vi "Angle.vi"() -> ()   [LabVIEW 2013]
uses:
  Robot Global Data.vi
panel:
  out "Angle":dbl
  in  "Samples Per Second":dbl=1000.0
  in  "Average Bits":u8=3 max=15
  out "Voltage Display":cluster{"Value":dbl, "Voltage":dbl}(graph)
  out "Average Voltage":dbl
  out "Voltage":dbl
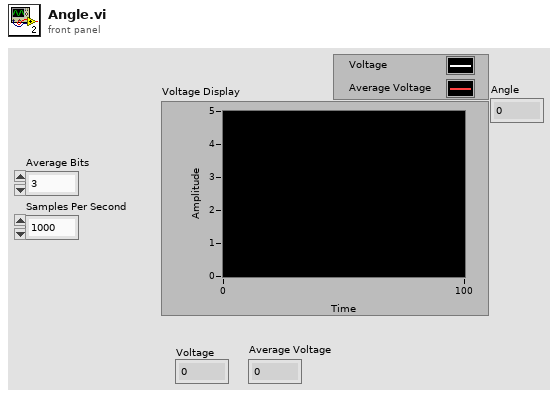
[diagram p1: front panel]
types:
  T1 = typedef "WPI_AnalogChannelDevRef.ctl" = cluster{"DevStatus":errorcluster, "Analog Module":T2, "Analog Channel":T3}
  T2 = typedef "FPGA_TypedefAnalogModule.ctl" = enum16{"Analog Module 1", "Analog Module 2"}
  T3 = typedef "FPGA_AIChannel.ctl" = enum8{"AI 1", "AI 2", "AI 3", "AI 4", "AI 5", "AI 6", "AI 7", "AI 8", "Invalid"}
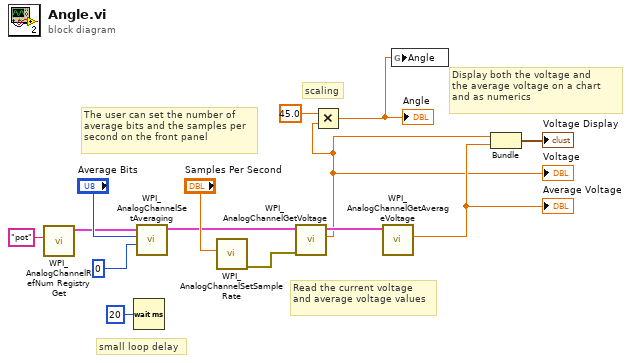
[diagram p0: block diagram]
diagram:
  # "scaling"
  # "small loop delay"
  # "Read the current voltage\nand average voltage values"
  # "Display both the voltage and\nthe average voltage on a chart\nand as numerics"
  # "The user can set the number of \naverage bits and the samples per\nsecond on the front panel"
  n1 = call <vilib>:"WPI_AnalogChannelRefNum Registry Get.vi"("refnum name"="pot") -> ("AIDeviceRef"=w5:T1)  [unwired: 9 in, 1 out]
  n2 = Wait (ms)(milliseconds to wait=u32 20) -> ()  [unwired: 1 out]
  n3 = call <vilib>:"WPI_AnalogChannelSetAveraging.vi"("OversampleBits"=u8 0, "AverageBits"="Average Bits", "AIDeviceRef"=w5) -> ("AIDeviceRef"=w7:T1)  [unwired: 1 in, 7 out]
  n4 = call <vilib>:"WPI_AnalogChannelSetSampleRate.vi"("Samples Per Second"="Samples Per Second") -> ("error out"=w6:errorcluster)  [unwired: 3 in, 7 out]
  n5 = call <vilib>:"WPI_AnalogChannelGetVoltage.vi"("error in (no error)"=w6, "AIDeviceRef"=w7) -> ("Voltage"=w3:dbl, "AIDeviceRef"=w14:T1)  [unwired: 8 out]
  "Voltage" <- w3
  n6 = Multiply(x=45.0, y=w3) -> (x*y=w1:dbl)
  "Angle" <- w1
  n7 = call <vilib>:"WPI_AnalogChannelGetAverageVoltage.vi"("AIDeviceRef"=w14) -> ("Voltage"=w13:dbl)  [unwired: 1 in, 9 out]
  "Average Voltage" <- w13
  n8 = global write "Robot Global Data.vi" "Angle"(w1) -> ()
  n9 = Bundle("Voltage"=w3, "Voltage"=w13) -> (→"Voltage Display":cluster{"Voltage":dbl, "Voltage":dbl})  [unwired: 1 out]
